vi "Estimate_State-Space_Model_from_FRFs_Parameter_Adjustment_v1.vi"() -> ()   [LabVIEW 2022 SP3]
doc: "This example demonstrates how to use frequency-domain data to estimate a state-space model. \n\n<B>Instructions:</B>\n1) Run this VI.\n2) Observe how the simulated frequency response matches the measured frequency response.\n3) Change the orders of the models, and observe how these changes affect the estimation error."
uses:
  <vilib>/addons/System Identification/Model Typedefs.llb/SI Pole-Zero Plot.ctl
  <vilib>/addons/System Identification/Frequency Domain Estimation.llb/SI Estimate Discrete State-Space Model from FRF (SISO Arbitrary).vi
  <vilib>/addons/System Identification/NI_SysID.lvlib
panel:
  in  "confidence level (%)":dbl=99.0 format="%_2f"
  out "pole-zero plot":T1
  in  "name or relative path":path=path "C:/Users/LAV-UFSC/OneDrive - UFSC/Documents/LAV - TCC/Dados-Experimentos/25-04/frf_2.txt"
  in  "noise subspace (%)":dbl=77.0
  in  "FRF format":T2={"dB on? (F)"=FALSE, "unwrap phase? (F)"=FALSE, "convert to degree? (F)"=TRUE}
  out "Phase Response":cluster{"frequency":dbl[], "amplitude":dbl[]}[](graph)
  out "Magnitude Response":cluster{"frequency":dbl[], "amplitude":dbl[]}[](graph)
  in  "Order":i32=67
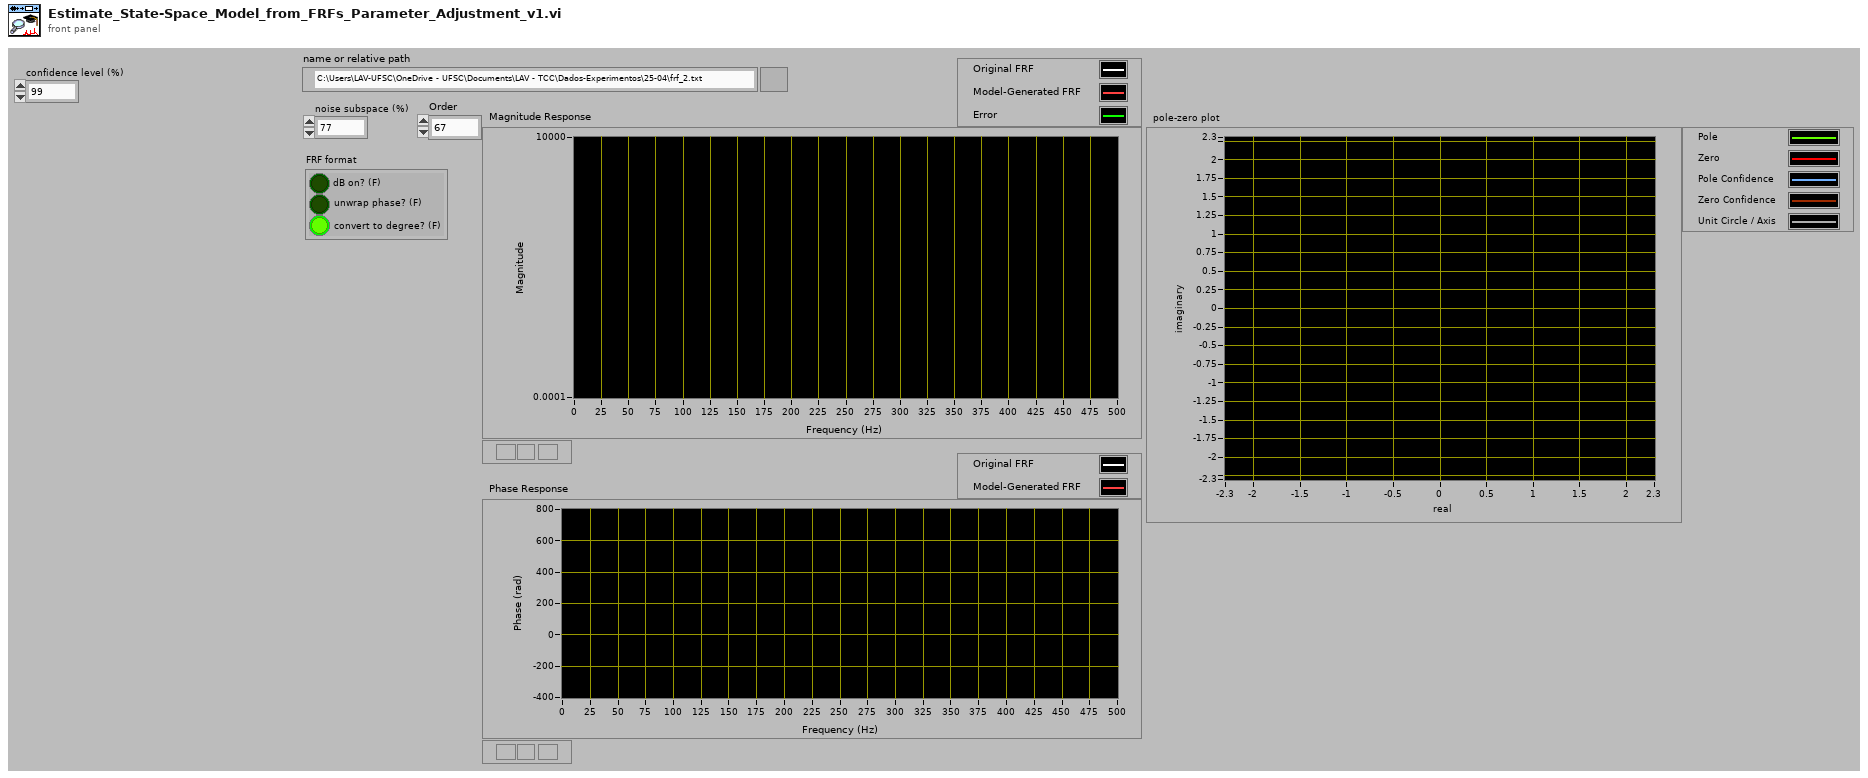
[diagram p1: front panel]
types:
  T1 = typedef "NI_SysID.lvlib/SI Pole-Zero Plot.ctl" = cluster{"frequency":dbl[], "amplitude":dbl[]}[]
  T2 = cluster{"dB on? (F)":bool, "unwrap phase? (F)":bool, "convert to degree? (F)":bool}
  T3 = cluster{"start frequency":dbl, "end frequency":dbl, "num of freq bins":i32, "interval type":u16}
  T4 = typedef "NI_SysID.lvlib/si_generic model.ctl" = cluster{"attributes":cluster{"version":string, "model type":T5, "input names":string[], "output names":string[], "notes":string}, "coefficients":cluster{"A ":dbl[][][], "B":dbl[][][], "F":dbl[][][], "C":dbl[][][], "D":dbl[][][]}, "std deviations":cluster{"A ":dbl[][][], "B":dbl[][][], "F":dbl[][][], "C":dbl[][][], "D":dbl[][][]}, "coefficients covariance":dbl[][][], "noise variance":dbl[][], "fs":dbl, "system info":cluster{"number of inputs":i32, "number of outputs":i32, "A order":i32[][], "B order":i32[][], "F order":i32[][], "C order":i32[][], "D order":i32[][], "Delays":i32[][]}, "kalman gain":dbl[][], "initial state":dbl[], "trans func":cluster{"betas":dbl[], "alphas":dbl[]}[][], "zeros-poles":cluster{"zeros":cdb[], "poles":cdb[], "gain":dbl}[][], "std of trans func":cluster{"betas":dbl[], "alphas":dbl[]}[][], "std of zeros-poles":cluster{"zeros":cdb[], "poles":cdb[], "gain":dbl}[][], "trans func (noise)":cluster{"betas":dbl[], "alphas":dbl[]}[][], "std of trans func (noise)":cluster{"betas":dbl[], "alphas":dbl[]}[][], "zeros-poles (noise)":cluster{"zeros":cdb[], "poles":cdb[], "gain":dbl}[][], "std of zeros-poles (noise)":cluster{"zeros":cdb[], "poles":cdb[], "gain":dbl}[][], "Symbolic State Space Model":cluster{"Symbolic A":string[][], "Symbolic B":string[][], "Symbolic C":string[][], "Symbolic D":string[][], "Symbolic K":string[][], "Symbolic Initial State":string[]}, "delay":dbl[][], "variables":T6, "grey trans func spec":cluster{"orders of TF model":cluster{" num order":i32, "den order":i32}, "# of zeros/poles at origin":cluster{"zeros/poles":u16, "number ":i32}, "delay initial?":bool, "gain initial?":bool}}
  T5 = typedef "NI_SysID.lvlib/SI Model Type.ctl" = u16
  T6 = typedef "NI_SysID.lvlib/si_variables.ctl" = cluster{"name":string, "initial guess":dbl, "upper limit":dbl, "lower limit":dbl, "value":dbl}[]
  T7 = typedef "NI_SysID.lvlib/si_Bode Phase Plot.ctl" = cluster{"frequency":dbl[], "amplitude":dbl[]}[]
  T8 = typedef "NI_SysID.lvlib/si_Bode Magnitude Plot.ctl" = cluster{"frequency":dbl[], "amplitude":dbl[]}[]
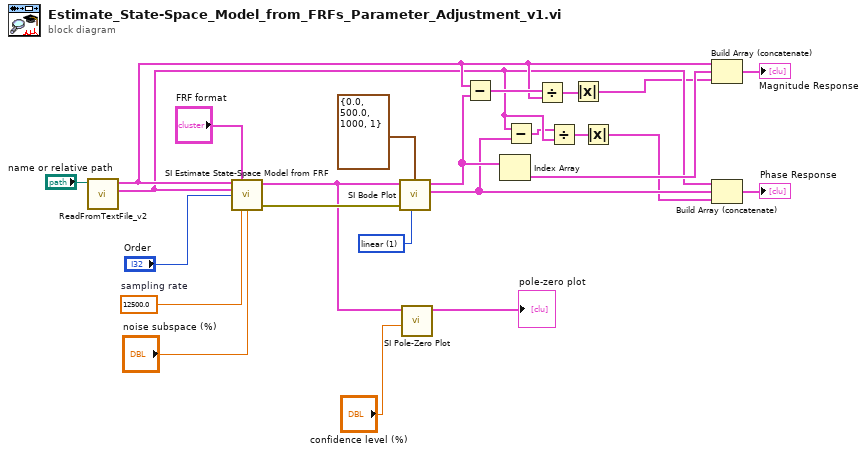
[diagram p0: block diagram]
diagram:
  w22 = 12500.0  # sampling rate
  w14 = u16 1 items=["dB", "linear"] ("magnitude unit")
  n1 = call "ReadFromTextFile_v2.vi"("name or relative path"="name or relative path") -> ("Phase"=w5:cluster{dbl[], dbl[]}, "Magnitude"=w7:cluster{dbl[], dbl[]})  [unwired: 6 in, 2 out]
  n2 = call-poly <vilib>:"SI Estimate State-Space Model from FRF.vi"("FRF magnitude"=w7, "FRF format"="FRF format", "FRF phase"=w5, "number of states"="Order", "sampling rate (Hz)"=w22, "noise subspace (%)"="noise subspace (%)") -> ("system model out"=w11:T4, "error out"=w15:errorcluster)  [unwired: 2 in, 6 out]
  n3 = call <vilib>:"SI Bode Plot.vi"("magnitude unit"=w14, "freq info"=T3 {"start frequency"=0.0, "end frequency"=500.0, "num of freq bins"=1000, "interval type"=1}, "error in (no error)"=w15, "system model"=w11) -> ("Bode phase plot"=w12:T7, "Bode magnitude plot"=w13:T8)  [unwired: 3 in, 3 out]
  n4 = call <vilib>:"SI Pole-Zero Plot.vi"("confidence level (%)"="confidence level (%)", "system model"=w11) -> ("pole-zero plot"=→"pole-zero plot":T1)  [unwired: 8 in, 1 out]
  n5 = Subtract(x=w7, y=w13) -> (x-y=w8:T8)
  n6 = Index Array(array=w13) -> (element=w21:cluster{"frequency":dbl[], "amplitude":dbl[]})  [unwired: 1 in]
  n7 = Subtract(x=w5, y=w12) -> (x-y=w4:T7)
  n8 = Divide(x=w8, y=w7) -> (x/y=w3:T8)
  n9 = Divide(x=w4, y=w5) -> (x/y=w6:T7)
  n10 = Absolute Value(x=w3) -> (abs(x)=w2:T8)
  n11 = Absolute Value(x=w6) -> (abs(x)=w1:T7)
  n12 = Build Array (concatenate)(w7, w21, w2) -> (→"Magnitude Response":T8)
  n13 = Build Array (concatenate)(w5, w12, w1) -> (→"Phase Response":T7)
